vi "Celcius to Farenheit.vi"() -> ()   [LabVIEW 2016]
panel:
  out "F":dbl(slide) scale=0.0..100.0
  out "C":dbl(slide) scale=0.0..100.0
  out "Farenheit":dbl
  in  "Celcius":dbl
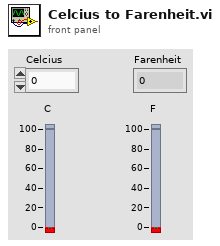
[diagram p1: front panel]
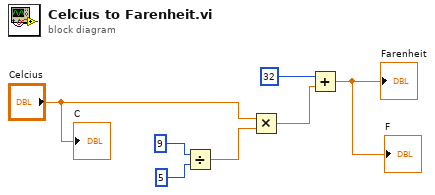
[diagram p0: block diagram]
diagram:
  n1 = Divide(x=9, y=5) -> (x/y=w5:dbl)
  n2 = Multiply(x="Celcius", y=w5) -> (x*y=w4:dbl)
  n3 = Add(x=32, y=w4) -> (x+y=→"Farenheit" →"F":dbl)
  "C" <- "Celcius"
